vi "Arrow_Teleop.vi"(11 "Joystick_Out":T1) -> ()   [LabVIEW 2020]
uses:
  Utility VIs/Joystick_Controls.ctl
  Subsystems/Arrow/Arrow_Cluster.ctl
  Subsystems/Arrow/Arrow_Control_States.ctl
  Globals/Arrow_Globals.vi
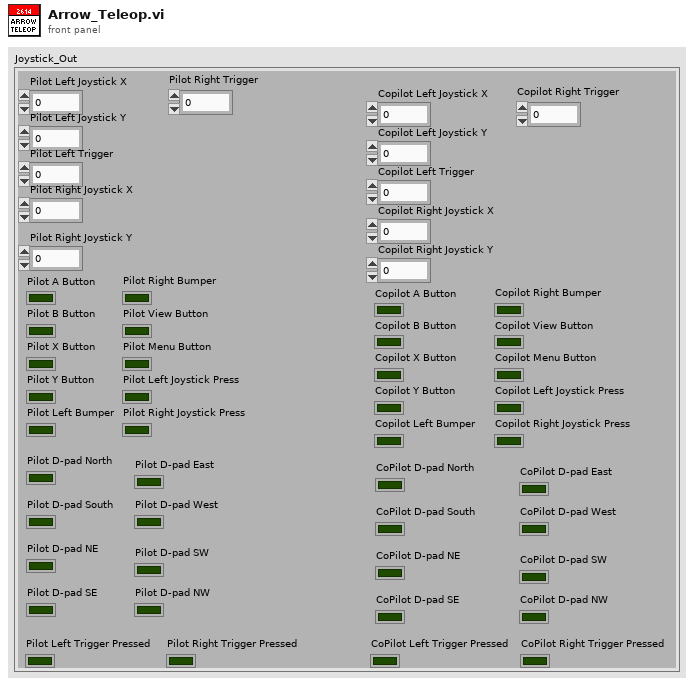
[diagram p1: front panel]
types:
  T1 = typedef "Joystick_Controls.ctl" = cluster{"Pilot Left Joystick X":dbl, "Pilot Left Joystick Y":dbl, "Pilot A Button":bool, "Pilot B Button":bool, "Pilot X Button":bool, "Pilot Y Button":bool, "Pilot Left Bumper":bool, "Pilot Right Bumper":bool, "Pilot View Button":bool, "Pilot Menu Button":bool, "Pilot Left Joystick Press":bool, "Pilot Right Joystick Press":bool, "Pilot Left Trigger":dbl, "Pilot Right Joystick X":dbl, "Pilot Right Joystick Y":dbl, "Pilot Right Trigger":dbl, "Copilot Left Joystick X":dbl, "Copilot Left Joystick Y":dbl, "Copilot A Button":bool, "Copilot B Button":bool, "Copilot X Button":bool, "Copilot Y Button":bool, "Copilot Left Bumper":bool, "Copilot Right Bumper":bool, "Copilot View Button":bool, "Copilot Menu Button":bool, "Copilot Left Joystick Press":bool, "Copilot Right Joystick Press":bool, "Copilot Left Trigger":dbl, "Copilot Right Joystick X":dbl, "Copilot Right Joystick Y":dbl, "Copilot Right Trigger":dbl, "Pilot D-pad North":bool, "Pilot D-pad South":bool, "Pilot D-pad East":bool, "Pilot D-pad West":bool, "Pilot D-pad NE ":bool, "Pilot D-pad SE":bool, "Pilot D-pad SW":bool, "Pilot D-pad NW":bool, "CoPilot D-pad North":bool, "CoPilot D-pad South":bool, "CoPilot D-pad East":bool, "CoPilot D-pad West":bool, "CoPilot D-pad NE":bool, "CoPilot D-pad SE":bool, "CoPilot D-pad SW":bool, "CoPilot D-pad NW":bool, "Pilot Left Trigger Pressed":bool, "Pilot Right Trigger Pressed":bool, "CoPilot Left Trigger Pressed":bool, "CoPilot Right Trigger Pressed":bool}
  T2 = typedef "Arrow_Cluster.ctl" = cluster{"Control_States":T3, "Manual_Throttle":dbl, "Angle_Goal":dbl}
  T3 = typedef "Arrow_Control_States.ctl" = enum16{"No-Op", "GoToAngle", "Manual_%Vbus"}
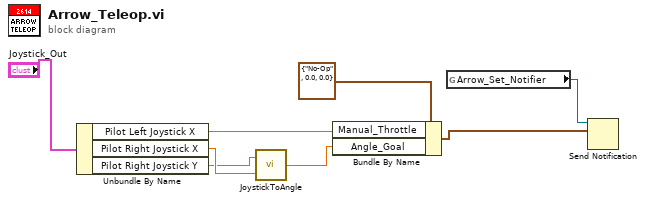
[diagram p0: block diagram]
diagram:
  n1 = Unbundle By Name("Joystick_Out") -> ("Pilot Left Joystick X"=w3:dbl, "Pilot Right Joystick X"=w5:dbl, "Pilot Right Joystick Y"=w4:dbl)
  n2 = call "JoystickToAngle.vi"("x"=w5, "y"=w4) -> ("theta"=w6:dbl)
  n3 = Bundle By Name(cluster=T2 {"Control_States"=enum."No-Op", "Manual_Throttle"=0.0, "Angle_Goal"=0.0}, "Manual_Throttle"=w3, "Angle_Goal"=w6) -> (w7:T2)
  n4 = global read "Arrow_Globals.vi" "Arrow_Set_Notifier"() -> (w8:refnum<notifier>)
  n5 = Send Notification(notification=w7, notifier=w8) -> ()  [unwired: 1 in, 2 out]
